vi "fastFrame_get_average.vi"(1 "array":dbl[][](array[numeric])) -> (4 "bg frames":dbl[][](array[numeric]), 6 "mol. frames":dbl[][](array[numeric]))   [LabVIEW 2012]
doc: "This Vi averages the frames for both the background and the molecular cycle and subtracts the background from the molecular signal in the time domain"
uses:
  global.vi
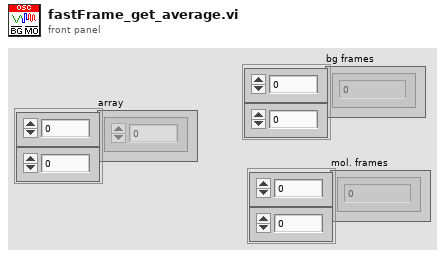
[diagram p1: front panel]
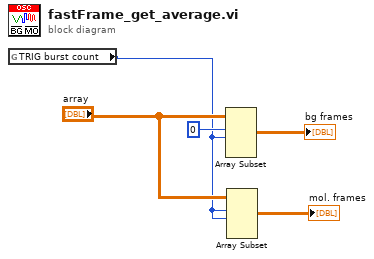
[diagram p0: block diagram]
diagram:
  n1 = global read "global.vi" "TRIG burst count"() -> (w2:i32)
  n2 = Array Subset(array="array", index (row)=0 ("index"), length (row)=w2) -> (→"bg frames":dbl[][])  [unwired: 2 in]
  n3 = Array Subset(array="array", index (row)=w2, length (row)=w2) -> (→"mol. frames":dbl[][])  [unwired: 2 in]
